vi "AMZ_S3_APIHLP_Convert Payer String to Enum.vi"(4 "Payer String":string) -> (1 "Payer":T1)   [LabVIEW 2015, in "LV Interface for Amazon S3.lvlib"]
doc: "Convert the Storage Class represented as a String to the Enum typedef representation."
uses:
  LV Interface for Amazon S3.lvlib
  Typedefs/AMZ_S3_Payer.ctl
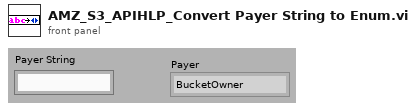
[diagram p1: front panel]
types:
  T1 = typedef "LV Interface for Amazon S3.lvlib/AMZ_S3_Payer.ctl" = enum16{"BucketOwner", "Requester"}
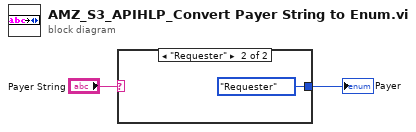
[diagram p0: block diagram]
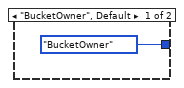
[diagram p2: hidden frame]
diagram:
  n1 = case shown="\"Requester\"" "Payer String" {
    tunnel: [AMZ_S3_Payer."BucketOwner" ("Payer") AMZ_S3_Payer."Requester" ("Payer")] -> w1
    frame "BucketOwner", Default {
    }
    frame "Requester" {
    }
  }
  "Payer" <- w1
